vi "SPI.vi"() -> ()   [LabVIEW 2021]
uses:
  <instrlib>/niDigital/niDigital.llb/niDigital Selected Function.ctl
  <instrlib>/niDigital/niDigital.llb/niDigital Get Site Results Site Numbers.vi
  <instrlib>/niDigital/niDigital.llb/niDigital Burst Pattern (Pass Fail).vi
panel:
  out "Site":string[](array[string])
  out "Pass?":bool[](array[boolean])
  in  "Simulate?":bool=TRUE
  in  "resource name":refnum<k15>="PXI1Slot2,PXI1Slot3"
  # "Overview\nThis getting started example demonstrates how to use the NI-Digital Pattern Driver API to load pre-created files with SPI pattern information on the NI Digital Pattern Instrument, burst the pattern, and record the site pass/fail information.\n\nInstructions\n1. Use the resource name control to select the digital pattern instrument. Ensure that the instrument name in the PinMap.pinmap file matches the resource name of the digital pattern instrument. The default value for the resource name is \"PXI1Slot2,PXI1Slot3\".\n2. Run the VI. The pattern pass/fail indicator displays results from each site.\n3. To run on hardware deselect simulate and modify the resource name as appropriate."
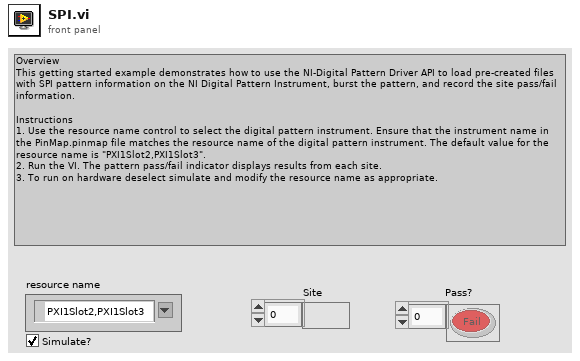
[diagram p1: front panel]
types:
  T1 = typedef "niDigital Selected Function.ctl" = i32
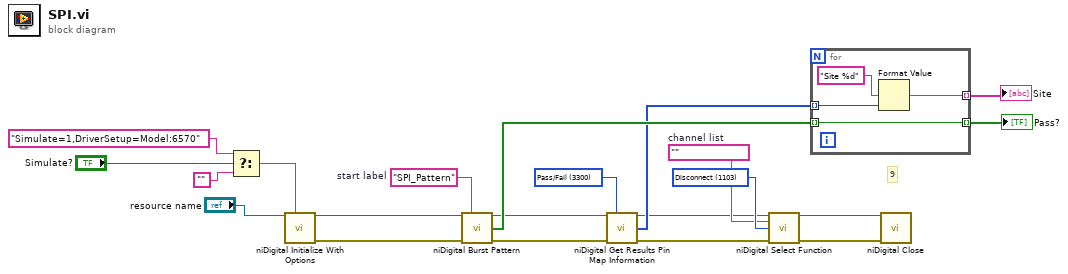
[diagram p0: block diagram]
diagram:
  w14 = ""  # channel list
  w15 = T1 1103 items=["Digital"=1100, "PPMU"=1101, "Off"=1102, "Disconnect"=1103] ("function")
  w20 = "SPI_Pattern"  # start label
  w16 = 3300 items=["Pass/Fail"=3300, "Capture Waveform"=3301] ("site result type")
  # "9"
  n1 = Select(t="Simulate=1,DriverSetup=Model:6570", s="Simulate?", f="") -> (s? t:f=w7:string)
  n2 = call <instrlib>:"niDigital Initialize With Options.vi"("resource name"="resource name", "option string"=w7) -> ("instrument handle"=w4:refnum<k15>, "error out"=w3:errorcluster)  [unwired: 12 in]
  n3 = call-poly <instrlib>:"niDigital Burst Pattern.vi"("instrument handle"=w4, "start label"=w20, "error in"=w3) -> ("instrument handle out"=w19:refnum<k15>, "pass"=w21:bool[], "error out"=w18:errorcluster)  [unwired: 10 in]
  n4 = call-poly <instrlib>:"niDigital Get Results Pin Map Information.vi"("instrument handle"=w19, "site result type"=w16, "error in"=w18) -> ("instrument handle out"=w13:refnum<k15>, "site numbers"=w17:i32[], "error out"=w12:errorcluster)  [unwired: 10 in]
  n5 = call <instrlib>:"niDigital Select Function.vi"("instrument handle"=w13, "channel list"=w14, "function"=w15, "error in"=w12) -> ("instrument handle out"=w10:refnum<k15>, "error out"=w11:errorcluster)  [unwired: 10 in]
  n6 = for {
    tunnel: w21 -> [w22] mode=indexing
    tunnel: w17 -> [w24] mode=indexing
    tunnel: [w23] -> w2 mode=indexing
    tunnel: [w22] -> w1 mode=indexing
    n7 = Format Value(format string="Site %d", value (0)=w24) -> (output string=w23:string)  [unwired: 1 in]
  }
  "Pass?" <- w1
  "Site" <- w2
  n8 = call <instrlib>:"niDigital Close.vi"("instrument handle"=w10, "error in"=w11) -> ()  [unwired: 13 in, 1 out]
